vi "Write Program.vi"(8 "error in (no error)":errorcluster, 10 "Program":string, 11 "SubParserConfig in":refnum<class "SubParserConfig.lvclass">) -> (0 "error out":errorcluster, 3 "SubParserConfig out":refnum<class "SubParserConfig.lvclass">)   [LabVIEW 2022 SP3, in "ArgumentParser.lvlib" / "SubParserConfig.lvclass"]
uses:
  SubParserConfig.lvclass
  SubParserConfig.lvclass/SubParserConfig.ctl
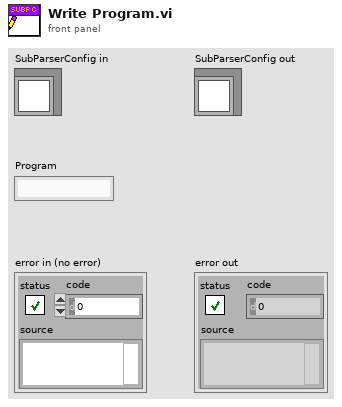
[diagram p1: front panel]
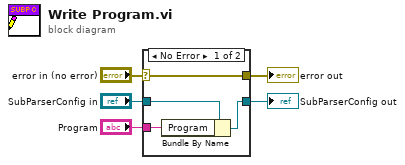
[diagram p0: block diagram]
diagram:
  n1 = case shown="No Error" "error in (no error)" {
    selector: "error in (no error)" -> [w9 w10]
    tunnel: [w9 w10] -> w4
    tunnel: [w7 w11] -> w2
    tunnel: "SubParserConfig in" -> [w8 w11]
    tunnel: "Program" -> [w6 _]
    frame No Error {
      n2 = Bundle By Name(cluster=w8, "Program"=w6) -> (w7:refnum<class "SubParserConfig.lvclass">)
    }
    frame Error {
    }
  }
  "error out" <- w4
  "SubParserConfig out" <- w2
